vi "Is Send VI.vi"(8 "error in (no error)":errorcluster, 11 "ProjectItem in":refnum<vi>) -> (0 "error out":errorcluster, 2 "Is Send VI?":bool, 3 "Path":path)   [LabVIEW 2020, in "Message Rescripter.lvlib"]
uses:
  Message Rescripter.lvlib
  <vilib>/Utility/traverseref.llb/TRef TravTarget.ctl
  <vilib>/Utility/traverseref.llb/VI Scripting - Traverse.lvlib
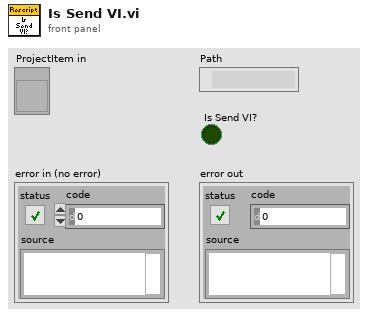
[diagram p1: front panel]
types:
  T1 = typedef "TRef TravTarget.ctl" = enum16{"FP", "BD", "Other"}
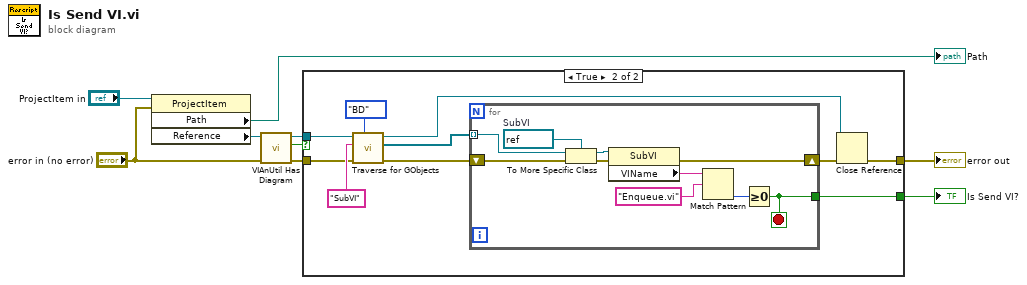
[diagram p0: block diagram]
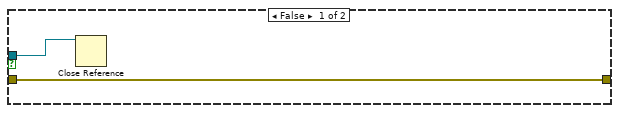
[diagram p2: hidden frame]
diagram:
  n1 = property class="ProjectItem"(reference="ProjectItem in", error in="error in (no error)") -> ("Path"=→"Path":path, "Reference"=w6:refnum<vi>)  [unwired: 2 out]
  n2 = call <vilib>:"VIAnUtil Has Diagram.vi"("error in (no error)"="error in (no error)", "VI in"=w6) -> ("error out"=w5:errorcluster, "Has Diag?"=w4:bool, "VI out"=w3:refnum<vi>)  [unwired: 4 in, 3 out]
  n3 = case shown="True" w4 {
    tunnel: w3 -> [w11 w19]
    tunnel: w5 -> [w10 w18]
    tunnel: [_ w15] -> w9
    tunnel: [w10 w14] -> w8
    frame False {
      n4 = Close Reference(reference=w11) -> ()  [unwired: 1 in, 1 out]
    }
    frame True {
      n5 = call <vilib>:"Traverse for GObjects.vi"("Traverse Target"=TRef_TravTarget."BD", "error in (no error)"=w18, "Class Name"="SubVI", "VI Refnum"=w19) -> ("error out"=w16:errorcluster, "References"=w13:refnum<vi>[], "dup VI Refnum"=w12:refnum<vi>)  [unwired: 4 in, 1 out]
      n6 = for {
        tunnel: w13 -> [w31] mode=indexing
        shift-right: [w30] -> w17
        shift-left: w16 -> [w28]
        tunnel: [w24] -> w15
        stop <- w24 stop-if-true
        w26 = refnum<vi> refnum  # SubVI
        n7 = To More Specific Class(target class=w26, reference=w31, error in=w28) -> (specific class reference=w29:refnum<vi>, error out=w27:errorcluster)
        n8 = property class="SubVI"(reference=w29, error in=w27) -> (error out=w30:errorcluster, "VIName"=w23:string)  [unwired: 1 out]
        n9 = Match Pattern(string=w23, regular expression="Enqueue.vi") -> (offset past match=w25:i32)  [unwired: 1 in, 3 out]
        n10 = Greater Or Equal To 0?(x=w25) -> (x >= 0?=w24:bool)
      }
      n11 = Close Reference(reference=w12, error in (no error)=w17) -> (error out=w14:errorcluster)
    }
  }
  "Is Send VI?" <- w9
  "error out" <- w8
